vi "Read Maximum speed.vi"(8 "error in (no error)":errorcluster, 11 "Motor-Analog in":refnum<class "Motor-Analog.lvclass">) -> (0 "error out":errorcluster, 2 "Maximum speed":dbl, 3 "Motor-Analog out":refnum<class "Motor-Analog.lvclass">)   [LabVIEW 2013, in "PowderDeposition.lvlib" / "Motor-Analog.lvclass"]
uses:
  Motor-Analog.lvclass
  Motor-Analog.lvclass/Motor-Analog.ctl
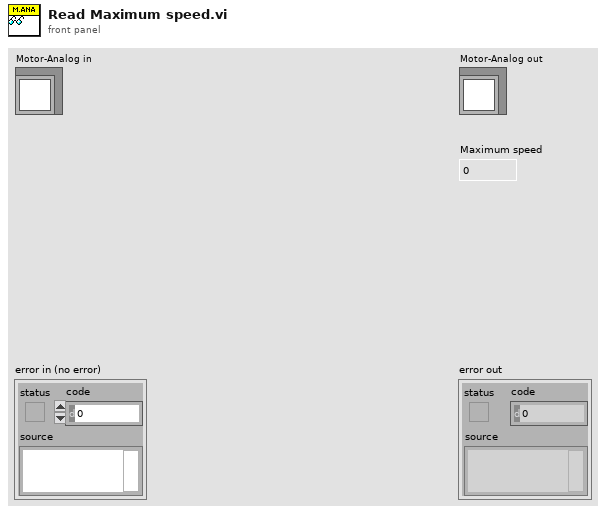
[diagram p1: front panel]
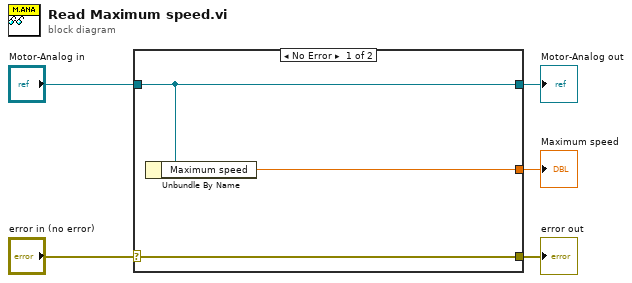
[diagram p0: block diagram]
diagram:
  n1 = case shown="No Error" "error in (no error)" {
    selector: "error in (no error)" -> [w8 w9]
    tunnel: [w8 w9] -> w4
    tunnel: [w7 w10] -> w2
    tunnel: "Motor-Analog in" -> [w7 w10]
    tunnel: [w6 _] -> w1
    frame No Error {
      n2 = Unbundle By Name(w7) -> ("Maximum speed"=w6:dbl)
    }
    frame Error {
    }
  }
  "error out" <- w4
  "Motor-Analog out" <- w2
  "Maximum speed" <- w1
